vi "File Page.vi"(8 "error in (no error)":errorcluster, 11 "Node Ptr":T1 format="%.0x") -> (0 "error out":errorcluster)   [LabVIEW 2019, in "Telemetry System Explorer.lvlib"]
uses:
  Telemetry System Explorer.lvlib
  <vilib>/NI VeriStand/Custom Device API/Custom Device API.lvlib
  <vilib>/NI VeriStand/Custom Device API/Custom Device Target Type.ctl
  Shared/Constants.vi
  Shared/Telemetry Shared.lvlib
  <vilib>/NI VeriStand/Custom Device API/Set Item Property (Boolean).vi
  <vilib>/NI VeriStand/Custom Device API/Set Item Property (String Array).vi
  <vilib>/NI VeriStand/Custom Device API/Custom Device Item Ref.ctl
panel:
  out "Example Log File Path":path
  in  "Timestamp":bool
  in  "Log File Directory":path
  in  "SHDocVw.IWebBrowser":refnum<k7>(container)
  in  "Specific Header":cluster{"Section Name":string}={"Section Name"="Specific Page Settings"}
  in  "General Header":cluster{"Section Name":string}={"Section Name"="General Page Settings"}
  in  "Description":string
  in  "Name":string
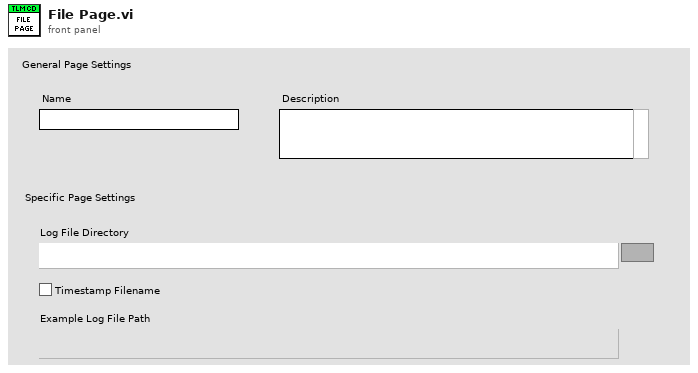
[diagram p1: front panel]
types:
  T1 = typedef "Custom Device API.lvlib/Custom Device Item Ref.ctl" = u64
  T2 = typedef "Custom Device API.lvlib/Custom Device Target Type.ctl" = enum16{"PharLap", "VxWorks", "Windows", "Linux_32_ARM", "Linux_x64"}
  T3 = typedef "Custom Device API.lvlib/Custom Device Commands.ctl" = enum16{"Default", "Item renamed", "Shutdown", "Dynamic button pressed"}
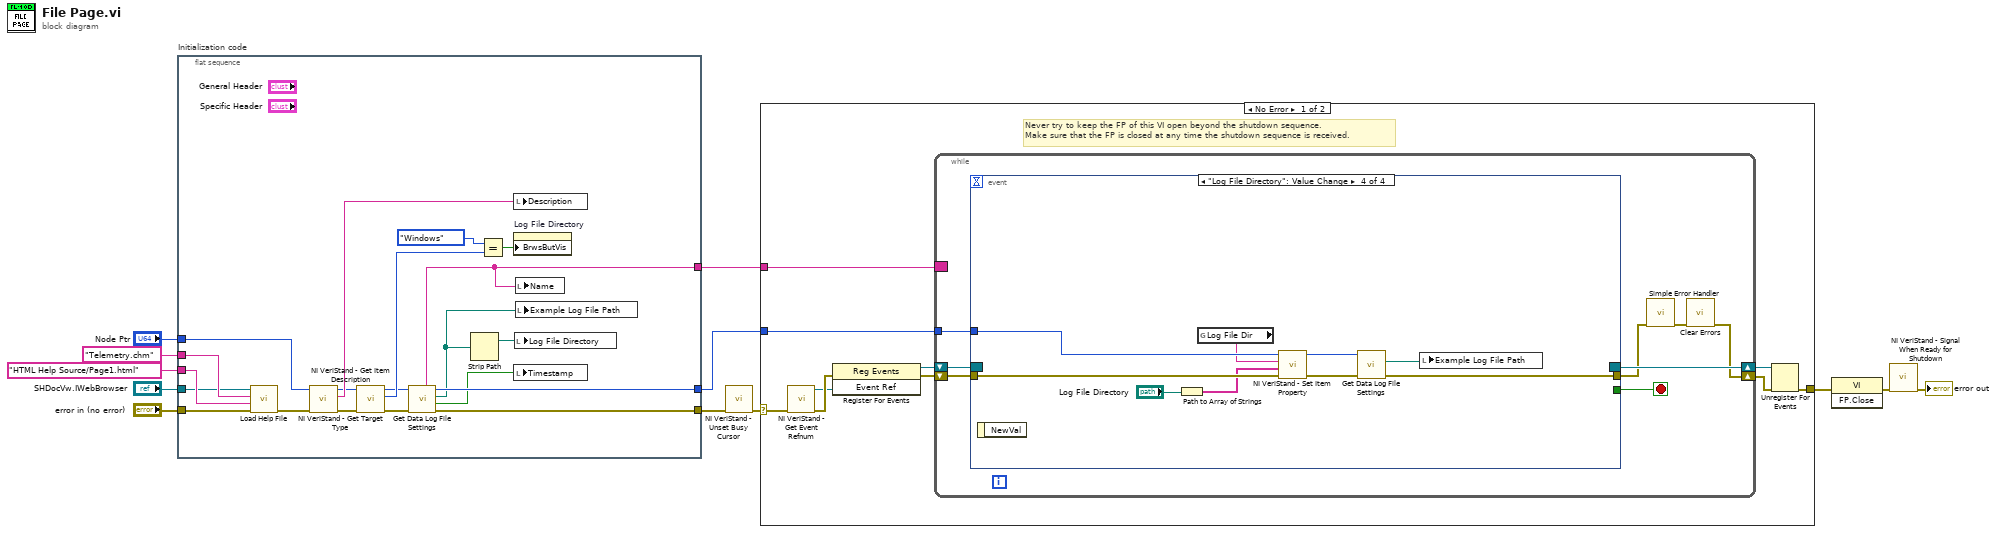
[diagram p0: block diagram]
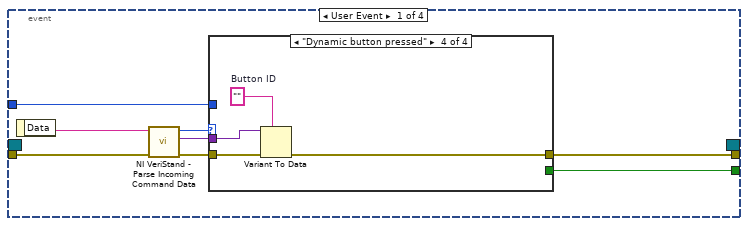
[diagram p2: hidden frame]
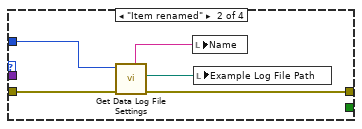
[diagram p4: hidden frame]
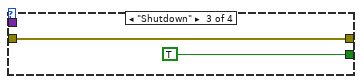
[diagram p5: hidden frame]
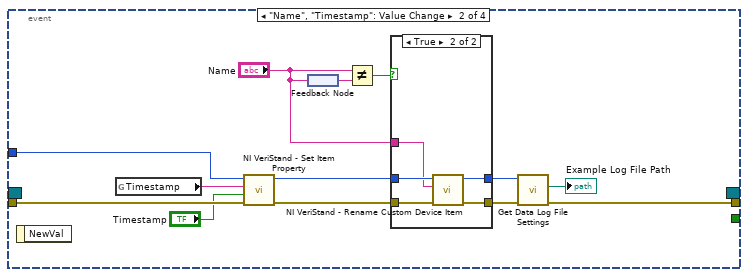
[diagram p6: hidden frame]
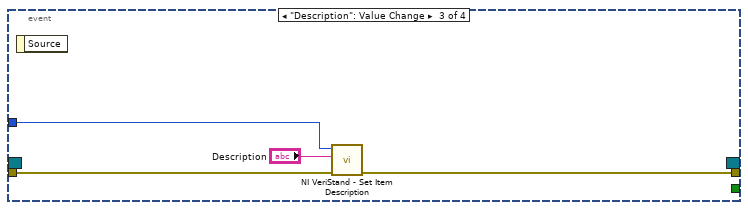
[diagram p8: hidden frame]
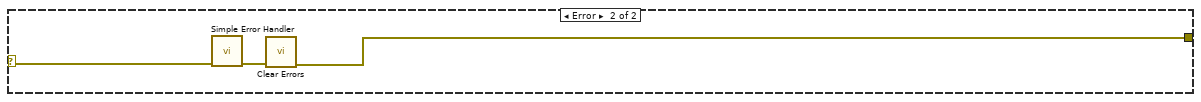
[diagram p9: hidden frame]
diagram:
  n1 = flat-sequence "Initialization code" {
    tunnel: "error in (no error)" -> [w29]
    tunnel: "Node Ptr" -> [w31]
    tunnel: [w17] -> w8
    tunnel: [w19] -> w5
    tunnel: "SHDocVw.IWebBrowser" -> [w25]
    tunnel: "HTML Help Source/Page1.html" ("CD_CHM_Section") -> [w27]
    tunnel: "Telemetry.chm" ("CD_CHM_FileName") -> [w26]
    tunnel: [w13] -> w1
    frame #0 {
      n2 = call "Load Help File.vi"("error in (no error)"=w29, "HTML File to Load"=w27, "Main CHM File"=w26, "Browser"=w25) -> ("error out"=w28:errorcluster)  [unwired: 7 in]
      n3 = call <vilib>:"NI VeriStand - Get Item Description.vi"("error in (no error)"=w28, "Item Ref in"=w31) -> ("error out"=w32:errorcluster, "Description"=w30:string, "Item Ref out"=w24:T1)  [unwired: 7 out]
      n4 = call <vilib>:"NI VeriStand - Get Target Type.vi"("error in (no error)"=w32, "Item Ref in"=w24) -> ("error out"=w18:errorcluster, "Target Type"=w21:T2, "Item Ref out"=w20:T1)  [unwired: 7 in]
      n5 = call "Get Data Log File Settings.vi"("error in (no error)"=w18, "File Ref In"=w20) -> ("error out"=w17:errorcluster, "Timestamp"=w14:bool, "File Path"=w15:path, "File Ref Out"=w19:T1, "Name"=w13:string)  [unwired: 5 in]
      n6 = Strip Path(path=w15) -> (stripped path=w16:path)  [unwired: 1 out]
      n7 = Equal?(x=Custom_Device_Target_Type."Windows" ("Target Type"), y=w21) -> (x = y?=w23:bool)
      n8 = local write "Description"(w30) -> ()
      n9 = property on="Log File Directory" class="Path"("BrwsButVis"=w23) -> ()  [unwired: 2 in, 2 out]
      n10 = local write "Timestamp"(w14) -> ()
      n11 = local write "Log File Directory"(w16) -> ()
      n12 = local write "Name"(w13) -> ()
      n13 = local write "Example Log File Path"(w15) -> ()
    }
  }
  n14 = call <vilib>:"NI VeriStand - Unset Busy Cursor.vi"("error in (no error)"=w8) -> ("error out"=w7:errorcluster)  [unwired: 10 out]
  n15 = case shown="No Error" w7 {
    selector: w7 -> [w34 w106]
    tunnel: [w39 w104] -> w12
    tunnel: w5 -> [w35 _]
    tunnel: w1 -> [w33 _]
    frame No Error {
      # "Never try to keep the FP of this VI open beyond the shutdown sequence.\nMake sure that the FP is closed at any time the shutdown sequence is received."
      n16 = call <vilib>:"NI VeriStand - Get Event Refnum.vi"("error in (no error)"=w34) -> ("error out"=w42:errorcluster, "Event Ref"=w38:refnum<user-event>)  [unwired: 9 out]
      n17 = register-events(error in=w42, w38) -> (reference out=w36:refnum<event-registration>, error out=w37:errorcluster)  [unwired: 1 in]
      n18 = while {
        tunnel: w35 -> [w46]
        shift-right: [w43] -> w40
        shift-left: w37 -> [w49]
        shift-right: [w50] -> w41
        shift-left: w36 -> [w48]
        border: w33 -> [_]
        stop <- w47 stop-if-true
        n19 = event shown="[3] \"Log File Directory\": Value Change" {
          selector: w48 -> [_ _ _ _]
          dyn-events: [_ _ _ _] -> w50
          timeout: _ -> [_ _ _ _]
          tunnel: w49 -> [w58 w83 w93 w102]
          tunnel: [w54 _ _ _] -> w47
          tunnel: [w53 w73 w92 w95] -> w45
          tunnel: w46 -> [w52 w81 w94 w101]
          event User Event {
            n20 = event-data() -> ("Data"=w57:string)  [unwired: 1 out]
            n21 = call <vilib>:"NI VeriStand - Parse Incoming Command Data.vi"("error in (no error)"=w58, "Incoming data"=w57) -> ("error out"=w56:errorcluster, "Outgoing data"=w51:variant, "Action"=w55:T3)  [unwired: 7 out]
            n22 = case shown="\"Dynamic button pressed\"" w55 {
              tunnel: w56 -> [w59 w64 w65 w70]
              tunnel: [_ _ TRUE _] -> w54
              tunnel: [w59 w63 w65 w67] -> w53
              tunnel: w52 -> [_ w60 _ _]
              tunnel: w51 -> [_ _ _ w69]
              frame "Default", Default {
              }
              frame "Item renamed" {
                n23 = call "Get Data Log File Settings.vi"("error in (no error)"=w64, "File Ref In"=w60) -> ("error out"=w63:errorcluster, "File Path"=w62:path, "Name"=w61:string)  [unwired: 5 in, 2 out]
                n24 = local write "Name"(w61) -> ()
                n25 = local write "Example Log File Path"(w62) -> ()
              }
              frame "Shutdown" {
              }
              frame "Dynamic button pressed" {
                w68 = ""  # Button ID
                n26 = Variant To Data(error in=w70, type=w68, Variant=w69) -> (error out=w67:errorcluster)  [unwired: 1 out]
              }
            }
          }
          event "Name", "Timestamp": Value Change {
            n27 = event-data() -> ()  [unwired: 2 out]
            n28 = global read "Constants.vi" "Timestamp"() -> (w76:string)
            n29 = call-poly <vilib>:"NI VeriStand - Set Item Property.vi"("error in (no error)"=w83, "Value"="Timestamp", "Property Name"=w76, "Item Ref in"=w81) -> ("error out"=w82:errorcluster, "Item Ref out"=w80:T1)  [unwired: 5 in, 1 out]
            n30 = feedback-in #1("Name") -> ()
            n31 = feedback #1() -> (w78:string)
            n32 = Not Equal?(x="Name", y=w78) -> (x != y?=w77:bool)
            n33 = case shown="True" w77 {
              tunnel: w82 -> [w85 w90]
              tunnel: [w85 w89] -> w74
              tunnel: w80 -> [w84 w88]
              tunnel: "Name" -> [_ w87]
              tunnel: [w84 w86] -> w72
              frame False {
              }
              frame True {
                n34 = call <vilib>:"NI VeriStand - Rename Custom Device Item.vi"("error in (no error)"=w90, "New Name"=w87, "Item Ref in"=w88) -> ("error out"=w89:errorcluster, "Item Ref out"=w86:T1)  [unwired: 1 in, 6 out]
              }
            }
            n35 = call "Get Data Log File Settings.vi"("error in (no error)"=w74, "File Ref In"=w72) -> ("error out"=w73:errorcluster, "File Path"=→"Example Log File Path":path)  [unwired: 5 in, 3 out]
          }
          event "Description": Value Change {
            n36 = event-data() -> ()  [unwired: 2 out]
            n37 = call <vilib>:"NI VeriStand - Set Item Description.vi"("error in (no error)"=w93, "Description"="Description", "Item Ref in"=w94) -> ("error out"=w92:errorcluster)  [unwired: 8 out]
          }
          event "Log File Directory": Value Change {
            n38 = event-data() -> ()  [unwired: 2 out]
            n39 = Path to Array of Strings(0:"Log File Directory") -> (2:w99:string[])  [unwired: 1 out]
            n40 = global read "Constants.vi" "Log File Dir"() -> (w100:string)
            n41 = call-poly <vilib>:"NI VeriStand - Set Item Property.vi"("error in (no error)"=w102, "Value"=w99, "Property Name"=w100, "Item Ref in"=w101) -> ("error out"=w98:errorcluster, "Item Ref out"=w97:T1)  [unwired: 5 in, 1 out]
            n42 = call "Get Data Log File Settings.vi"("error in (no error)"=w98, "File Ref In"=w97) -> ("error out"=w95:errorcluster, "File Path"=w96:path)  [unwired: 5 in, 3 out]
            n43 = local write "Example Log File Path"(w96) -> ()
          }
        }
        n44 = call <vilib>:"Simple Error Handler.vi"("error in (no error)"=w45) -> ("error out"=w44:errorcluster)  [unwired: 1 in, 7 out]
        n45 = call <vilib>:"Clear Errors.vi"("error in (no error)"=w44) -> ("error out"=w43:errorcluster)  [unwired: 1 in, 5 out]
      }
      n46 = Unregister For Events(event registration refnum=w41, error in=w40) -> (error out=w39:errorcluster)
    }
    frame Error {
      n47 = call <vilib>:"Simple Error Handler.vi"("error in (no error)"=w106) -> ("error out"=w105:errorcluster)  [unwired: 1 in, 7 out]
      n48 = call <vilib>:"Clear Errors.vi"("error in (no error)"=w105) -> ("error out"=w104:errorcluster)  [unwired: 1 in, 5 out]
    }
  }
  n49 = invoke class="VI" method="FP.Close"(error in=w12) -> (error out=w11:errorcluster)  [unwired: 2 in, 2 out]
  n50 = call <vilib>:"NI VeriStand - Signal When Ready for Shutdown.vi"("error in (no error)"=w11) -> ("error out"=→"error out":errorcluster)  [unwired: 10 out]
